vi "Construct Topic.vi"(5 "Framework Instance Alias":string, 7 "Event Log Instance":refnum<class "LoggerReference.lvclass">, 8 "Lock Owner ID (\"\" = NOT Locked)":string, 9 "New Topic Data":variant, 10 "Name":string, 11 "Use Type Input As Initial Value?":bool) -> (0 "error out":errorcluster, 3 "Topic out":refnum<class "Topic.lvclass">)   [LabVIEW 2017, in "Mediator.lvlib" / "Topic.lvclass"]
doc: "<License>\nCopyright © 2017 Composed Systems, LLC | All rights reserved\nwww.composed.io\n\nAuthor: Ethan Stern <ethan.stern@composed.io>\n\nThis software is provided \"AS IS\" WITHOUT WARRANTIES, either express or implied, AND IS FOR EDUCATIONAL PURPOSES ONLY.\n</License>"
uses:
  Topic.lvclass
  gpm_packages/@cs/event-logger/Source/Composed Log/LoggerReference/LoggerReference.lvclass
  Topic.lvclass/Topic.ctl
  gpm_packages/@cs/variant/Source/VariantExtensions.lvlib
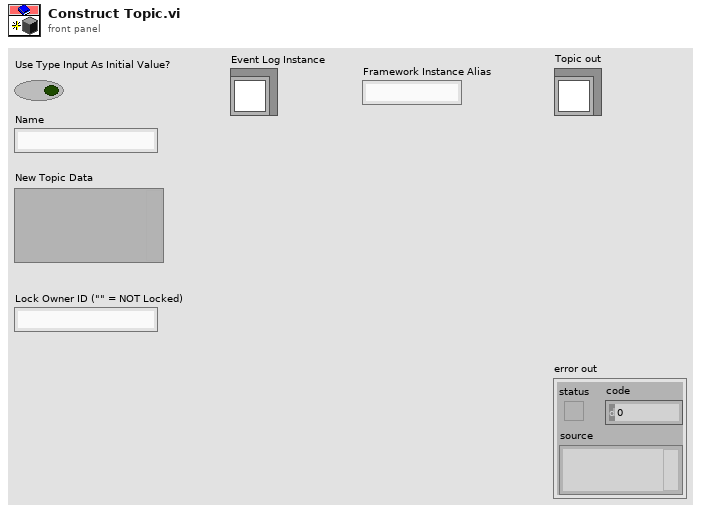
[diagram p1: front panel]
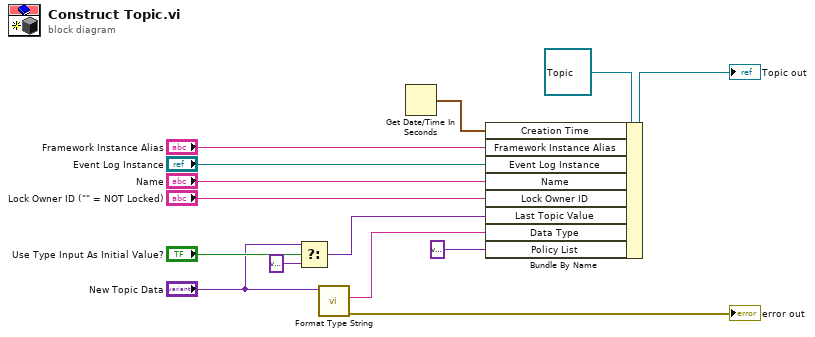
[diagram p0: block diagram]
diagram:
  n1 = Select(t="New Topic Data", s="Use Type Input As Initial Value?", f=variant) -> (s? t:f=w6:variant)
  n2 = call "Format Type String.vi"("Data Type"="New Topic Data") -> ("error out"=→"error out":errorcluster, "Type Name"=w11:string)  [unwired: 9 in]
  n3 = Get Date/Time In Seconds() -> (seconds since 1Jan1904=w1:timestamp)
  n4 = Bundle By Name(cluster=refnum<class "Topic.lvclass"> refnum ("Topic in"), "Creation Time"=w1, "Framework Instance Alias"="Framework Instance Alias", "Event Log Instance"="Event Log Instance", "Name"="Name", "Lock Owner ID"="Lock Owner ID (\"\" = NOT Locked)", "Last Topic Value"=w6, "Data Type"=w11, "Policy List"=variant ("Subscriber List")) -> (→"Topic out":refnum<class "Topic.lvclass">)
